vi "Get first target IP.vi"(8 "error in (no error)":errorcluster, 11 "System Definition File":path) -> (0 "error out":errorcluster, 3 "IPAddress":string)   [LabVIEW 2010, in "CAN Log Transfer and Convert.lvlib"]
uses:
  NationalInstruments.VeriStand.SystemDefinitionAPI
  CAN Log Transfer and Convert.lvlib
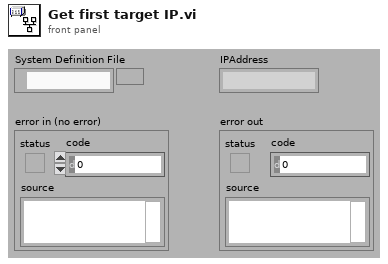
[diagram p1: front panel]
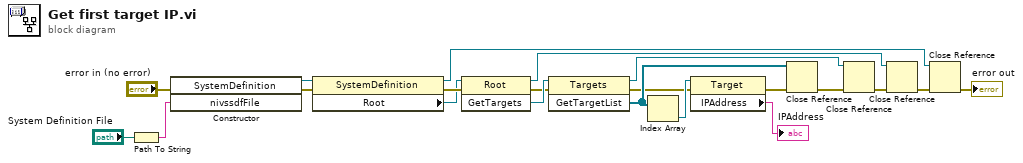
[diagram p0: block diagram]
diagram:
  n1 = Path To String(path="System Definition File") -> (string=w5:string)
  n2 = constructor class="SystemDefinition"(error in="error in (no error)", "nivssdfFile"=w5) -> (reference out=w2:refnum<k24>, error out=w3:errorcluster)  [unwired: 2 in, 2 out]
  n3 = property class="SystemDefinition"(reference=w2, error in=w3) -> (reference out=w20:refnum<k24>, error out=w11:errorcluster, "Root"=w10:refnum<k24>)
  n4 = invoke class="Root" method="GetTargets"(reference=w10, error in=w11) -> (reference out=w19:refnum<k24>, error out=w12:errorcluster, "GetTargets"=w13:refnum<k24>)  [unwired: 1 in]
  n5 = invoke class="Targets" method="GetTargetList"(reference=w13, error in=w12) -> (reference out=w18:refnum<k24>, error out=w1:errorcluster, "GetTargetList"=w17:refnum<k24>[])  [unwired: 1 in]
  n6 = Index Array(array=w17) -> (element=w15:refnum<k24>)  [unwired: 1 in]
  n7 = property class="Target"(reference=w15, error in=w1) -> (error out=w16:errorcluster, "IPAddress"=→"IPAddress":string)  [unwired: 1 out]
  n8 = Close Reference(reference=w17, error in (no error)=w16) -> (error out=w9:errorcluster)
  n9 = Close Reference(reference=w18, error in (no error)=w9) -> (error out=w8:errorcluster)
  n10 = Close Reference(reference=w19, error in (no error)=w8) -> (error out=w7:errorcluster)
  n11 = Close Reference(reference=w20, error in (no error)=w7) -> (error out=→"error out":errorcluster)
